vi "Clear Sessions.vi"(8 "error in (no error)":errorcluster, 11 "Session Handle in":T1) -> (0 "error out":errorcluster, 3 "Session Handle out":T1)   [LabVIEW 2015, in "Oil.lvclass"]
uses:
  Oil.lvclass
  Typedefs/Session Handle.ctl
  Oil.lvclass/Oil.ctl
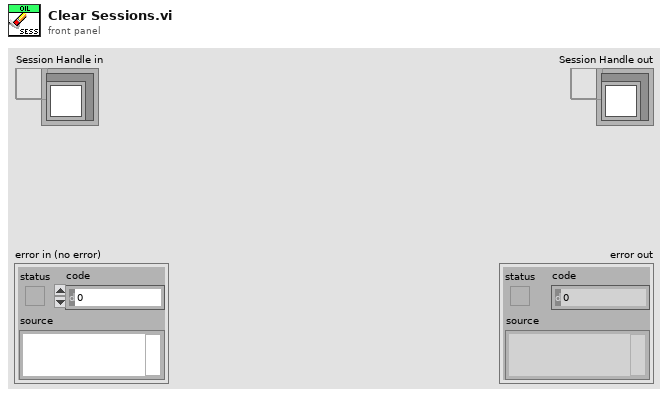
[diagram p1: front panel]
types:
  T1 = typedef "Oil.lvclass/Session Handle.ctl" = refnum<data-value>
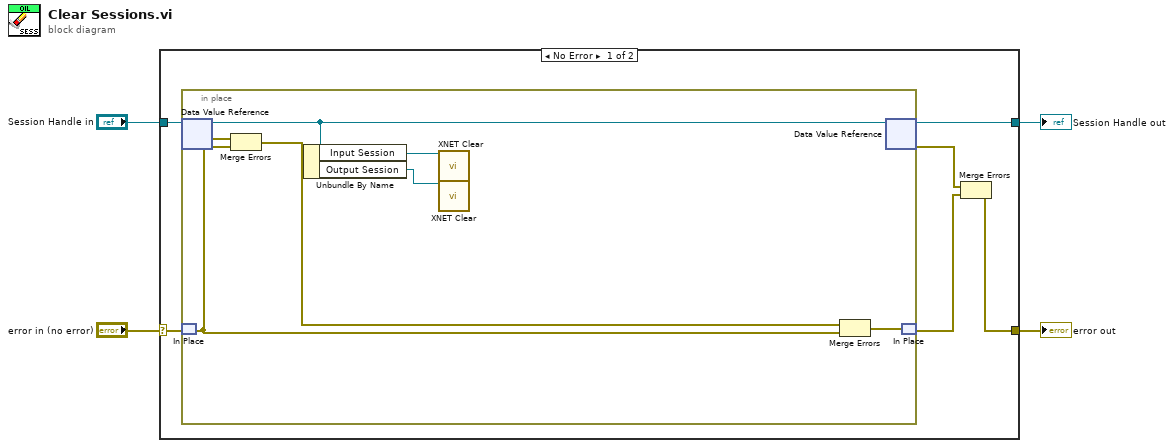
[diagram p0: block diagram]
diagram:
  n1 = case shown="No Error" "error in (no error)" {
    selector: "error in (no error)" -> [w5 w18]
    tunnel: "Session Handle in" -> [w10 w19]
    tunnel: [w9 w19] -> w3
    tunnel: [w6 w18] -> w2
    frame No Error {
      n2 = in-place {
        n3 = in-place-dvr #1(w10) -> (w11:refnum<class "Oil.lvclass">, w17:errorcluster)
        n4 = in-place-match #2(w5) -> (w15:errorcluster)
        n5 = Merge Errors(w15, w17) -> (w14:errorcluster)
        n6 = Unbundle By Name(w11) -> ("Input Session"=w13:refnum<k21>, "Output Session"=w12:refnum<k21>)
        n7 = call <vilib>:"XNET Clear.vi"("session in"=w13) -> ()  [unwired: 14 in, 1 out]
        n8 = call <vilib>:"XNET Clear.vi"("session in"=w12) -> ()  [unwired: 14 in, 1 out]
        n9 = Merge Errors(w14, w15) -> (w16:errorcluster)
        n10 = in-place-dvr #1(w11) -> (w9:T1, w7:errorcluster)
        n11 = in-place-match #2(w16) -> (w8:errorcluster)
      }
      n12 = Merge Errors(w7, w8) -> (w6:errorcluster)
    }
    frame Error {
    }
  }
  "Session Handle out" <- w3
  "error out" <- w2
